vi "SRV_Read_Comm.vi"(8 "error in (no error)":errorcluster, 10 "TCP Settings":T1={"Method"=enum."General", "bytes to read"=2000, "timeout ms (1000)"=1000}, 11 "SRV In":refnum<k5>) -> (0 "error out":errorcluster, 2 "Data out":string, 3 "SRV Out":refnum<k5>)   [LabVIEW 2009]
doc: "Reads data from the SRV.\n\n\nWritten for Benilde St. Margaret's School - Tim Jump\nBy Doug Schmertman - Logic PD\nCopyright 2012"
uses:
  TCP_Communication/SRV_TCP Settings.ctl
  TCP_Communication/SRV_Package Methods.ctl
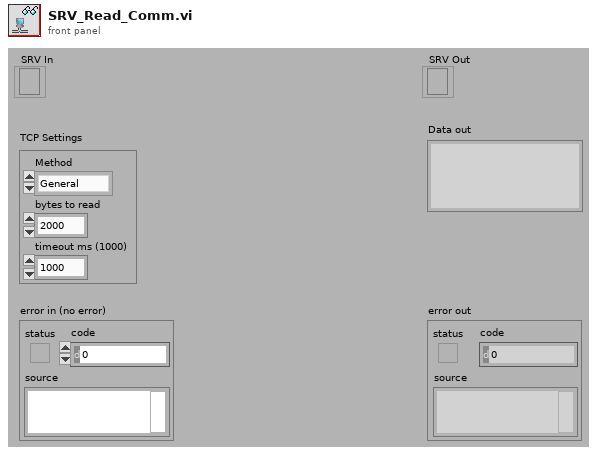
[diagram p1: front panel]
types:
  T1 = typedef "SRV_TCP Settings.ctl" = cluster{"Method":T2, "bytes to read":i32, "timeout ms (1000)":i32}
  T2 = typedef "SRV_Package Methods.ctl" = enum16{"General", "Standard", "CRLF", "Image", "HTML"}
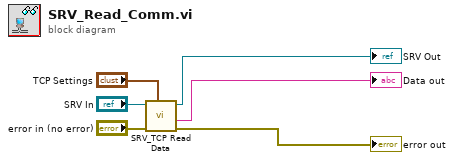
[diagram p0: block diagram]
diagram:
  n1 = call "SRV_TCP Read Data.vi"("TCP Settings"="TCP Settings", "error in"="error in (no error)", "connection ID in"="SRV In") -> ("error out"=→"error out":errorcluster, "data out"=→"Data out":string, "connection ID"=→"SRV Out":refnum<k5>)  [unwired: 2 in, 1 out]
